vi "波动性均值.vi"(1 "波动性表格":string[][](table)) -> (0 "波动性表格1":string[][](array[string]))   [LabVIEW 2015]
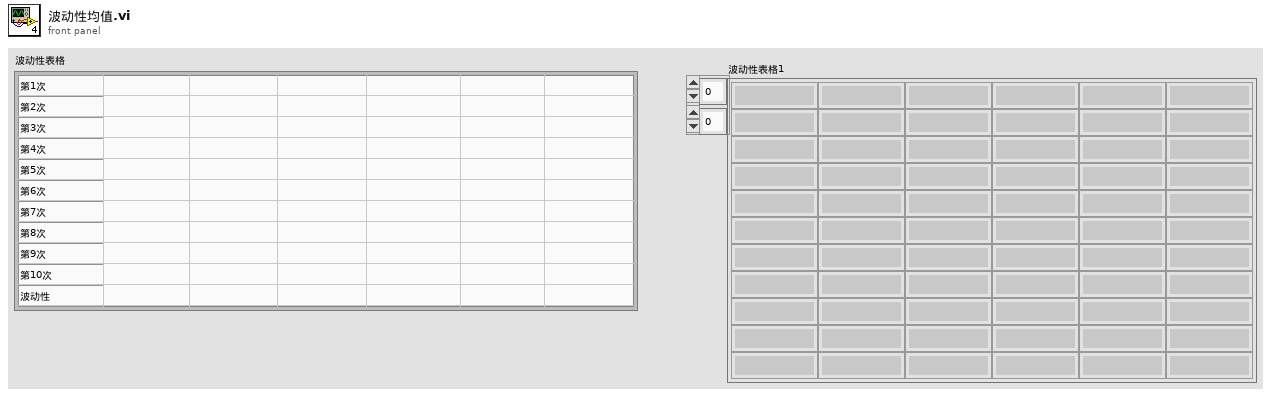
[diagram p1: front panel]
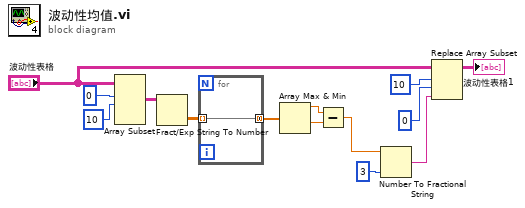
[diagram p0: block diagram]
diagram:
  n1 = Array Subset(array="波动性表格", index (row)=0 ("索引 (行)"), length (row)=10 ("索引 (行)")) -> (w7:string[][])  [unwired: 2 in]
  n2 = Fract/Exp String To Number(string=w7) -> (number=w12:dbl[][])  [unwired: 3 in, 1 out]
  n3 = for {
    tunnel: w12 -> [w15] mode=indexing
    tunnel: [w15] -> w4 mode=concatenating
  }
  n4 = Array Max & Min(array=w4) -> (max value=w3:dbl, min value=w2:dbl)  [unwired: 2 out]
  n5 = Subtract(x=w3, y=w2) -> (x-y=w1:dbl)
  n6 = Number To Fractional String(number=w1, precision (6)=i16 3 ("精度(6)")) -> (F-format string=w11:string)  [unwired: 2 in]
  n7 = Replace Array Subset(array="波动性表格", new element=w11, index (row)=10 ("索引 (行)"), index (col)=0 ("索引 (行)")) -> (→"波动性表格1":string[][])
